vi "AutoPilot.vi"(3 "Human Contribution":dbl, 4 "Drive Direction":dbl) -> (0 "End Contribution":dbl)   [LabVIEW 2018]
uses:
  SensorReadings.vi
panel:
  in  "Plot PID":bool
  out "PID Tracking":cluster{"Goal Wheel Position":dbl, dbl}(graph)={"Goal Wheel Position"=0.0, -6.7188720703125}
  out "Contribution Tracking":cluster{dbl, dbl, dbl}(graph)={0.335943603515625, 0.10438529174803275, -0.0}
  in  "Autopilot Deadband (deg)":dbl=1.0
  in  "Kp Butterfly":dbl=0.06
  in  "Ki Butterfly":dbl=0.01
  in  "Kd Butterfly":dbl
  in  "N-Diff Butterfly":i32=10
  in  "N-Int Butterfly":i32=25
  in  "Kf Butterfly":dbl=0.1
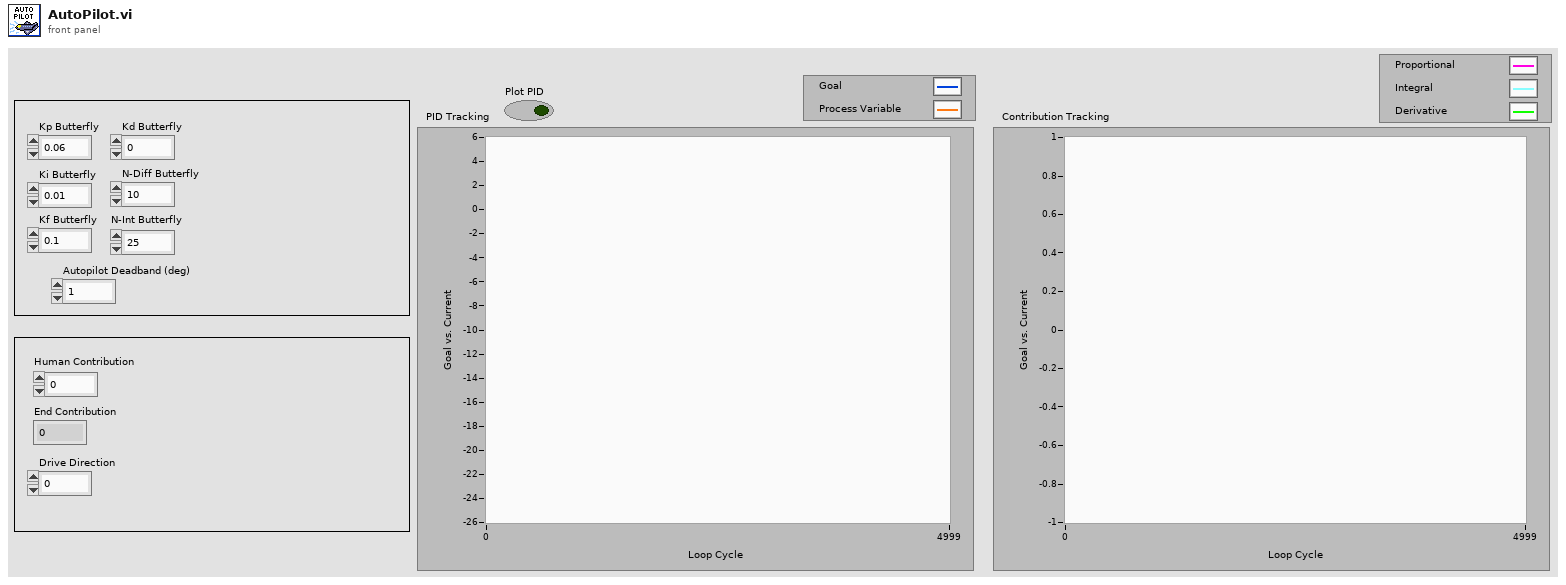
[diagram p1: front panel]
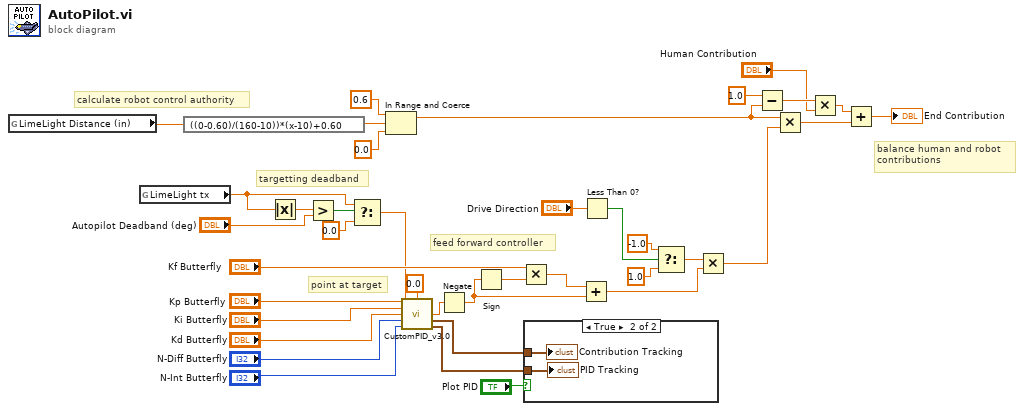
[diagram p0: block diagram]
diagram:
  # "point at target"
  # "calculate robot control authority"
  # "balance human and robot\ncontributions"
  # "targetting deadband"
  # "feed forward controller"
  n1 = global read "SensorReadings.vi" "LimeLight Distance (in)"() -> (w29:dbl)
  n2 = global read "SensorReadings.vi" "LimeLight tx"() -> (w15:dbl)
  n3 = expression code="((0-0.60)/(160-10))*(x-10)+0.60"(w29) -> (w28:dbl)
  n4 = Absolute Value(x=w15) -> (abs(x)=w17:dbl)
  n5 = Greater?(x=w17, y="Autopilot Deadband (deg)") -> (0:w16:bool)
  n6 = Select(t=w15, s=w16, f=0.0) -> (s? t:f=w14:dbl)
  n7 = In Range and Coerce(upper limit=0.6, x=w28, lower limit=0.0) -> (coerced(x)=w25:dbl)  [unwired: 1 out]
  n8 = call "CustomPID_v3.0.vi"("Kp"="Kp Butterfly", "Process Variable"=w14, "Goal"=0.0, "Ki"="Ki Butterfly", "Kd"="Kd Butterfly", "N-Diff"="N-Diff Butterfly", "N-Int"="N-Int Butterfly") -> ("Command"=w20:dbl, "Contribution Tracking"=w33:cluster{dbl, dbl, dbl}, "PID Tracking"=w34:cluster{"Goal Wheel Position":dbl, dbl})  [unwired: 5 in, 1 out]
  n9 = Negate(x=w20) -> (-x=w18:dbl)
  n10 = Sign(1:w18) -> (0:w19:dbl)
  n11 = Multiply(x="Kf Butterfly", y=w19) -> (x*y=w21:dbl)
  n12 = case shown="True" "Plot PID" {
    tunnel: w34 -> [_ w40]
    tunnel: w33 -> [_ w39]
    frame False {
    }
    frame True {
      "PID Tracking" <- w40
      "Contribution Tracking" <- w39
    }
  }
  n13 = Add(x=w21, y=w18) -> (x+y=w4:dbl)
  n14 = Less Than 0?(x="Drive Direction") -> (x < 0?=w3:bool)
  n15 = Select(t=-1.0, s=w3, f=1.0) -> (s? t:f=w6:dbl)
  n16 = Multiply(x=w6, y=w4) -> (x*y=w5:dbl)
  n17 = Subtract(x=1.0, y=w25) -> (x-y=w26:dbl)
  n18 = Multiply(x=w25, y=w5) -> (x*y=w30:dbl)
  n19 = Multiply(x=w26, y="Human Contribution") -> (x*y=w31:dbl)
  n20 = Add(x=w31, y=w30) -> (x+y=→"End Contribution":dbl)
